vi "Test Parsing Simple Example Whlie Loop Some Operations 1.vi"() -> ()   [LabVIEW 2014]
uses:
  <vilib>/Utility/traverseref.llb/TRef TravTarget.ctl
  <vilib>/Utility/traverseref.llb/VI Scripting - Traverse.lvlib
panel:
  out "WhileLoop code chunks":T1
  out "Array 2":string[](array[string])
  out "error out":errorcluster
  out "SubVI C calls":string[](array[string])
  out "error wires info":T2
  in  "vi path":path=path "C:/Users/lubo/Documents/LabView/LabVIEW-Universal-Transcriptor/Test/Examples For Parsing/Example While Loop Some Operations 1.vi"
  # "This is here just for debug, for now I'm going to scan error wires and transcript VI on it to some C call functions."
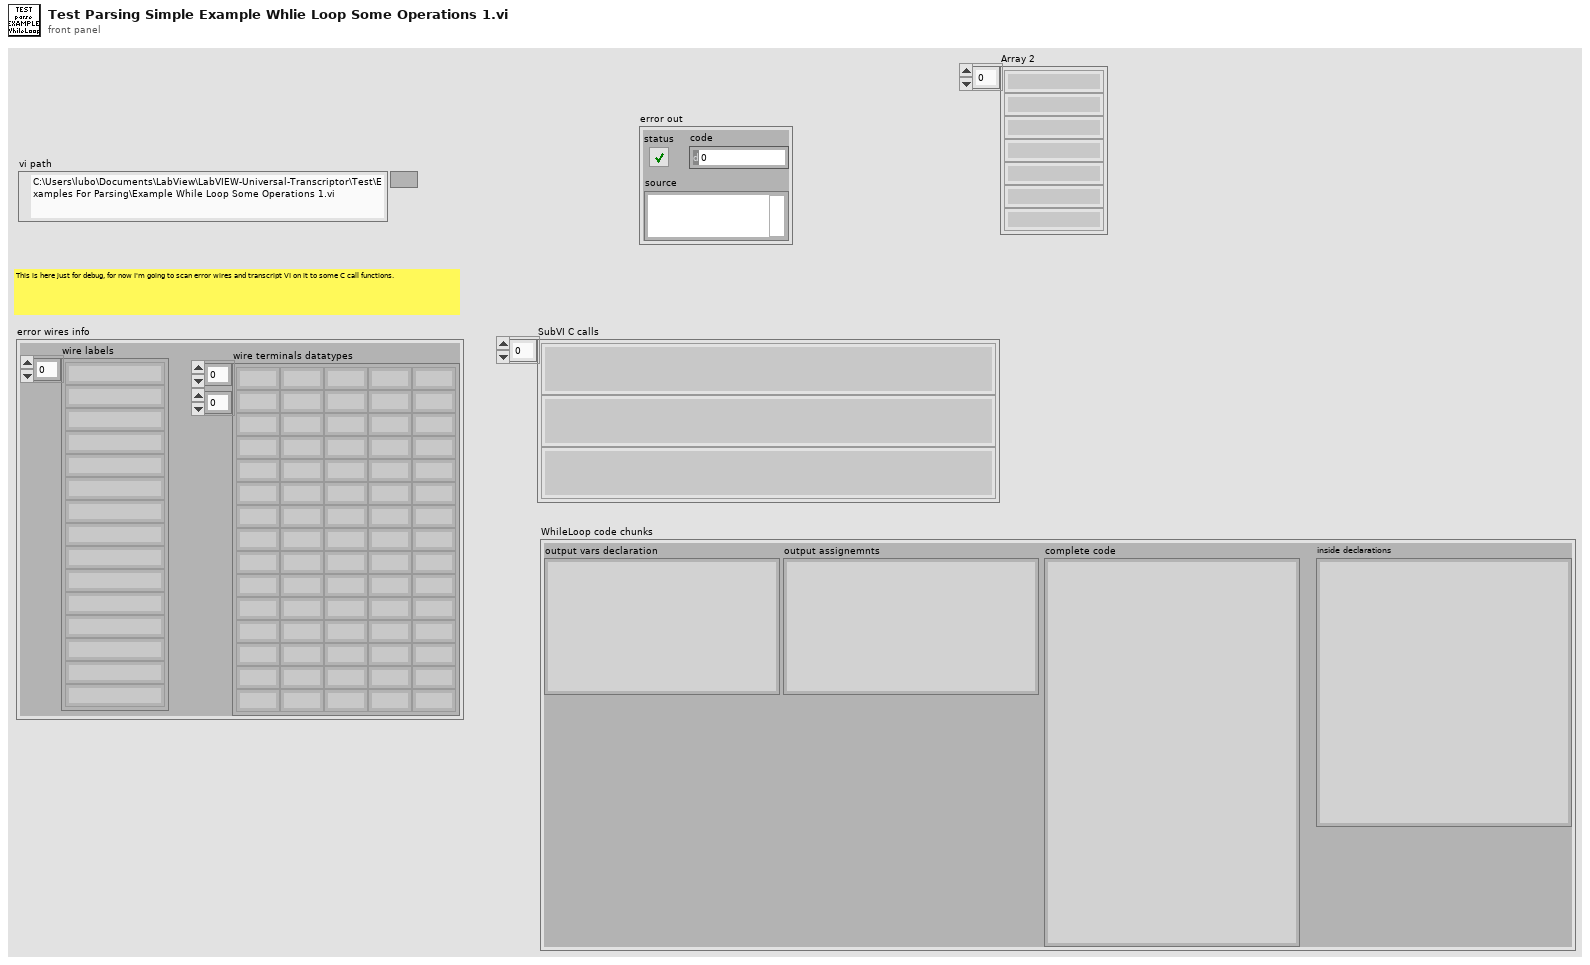
[diagram p1: front panel]
types:
  T1 = cluster{"output vars declaration":string, "output assignemnts":string, "complete code":string, "inside declarations":string}
  T2 = cluster{"wire labels":string[], "wire terminals datatypes":string[][]}
  T3 = typedef "TRef TravTarget.ctl" = enum16{"FP", "BD", "Other"}
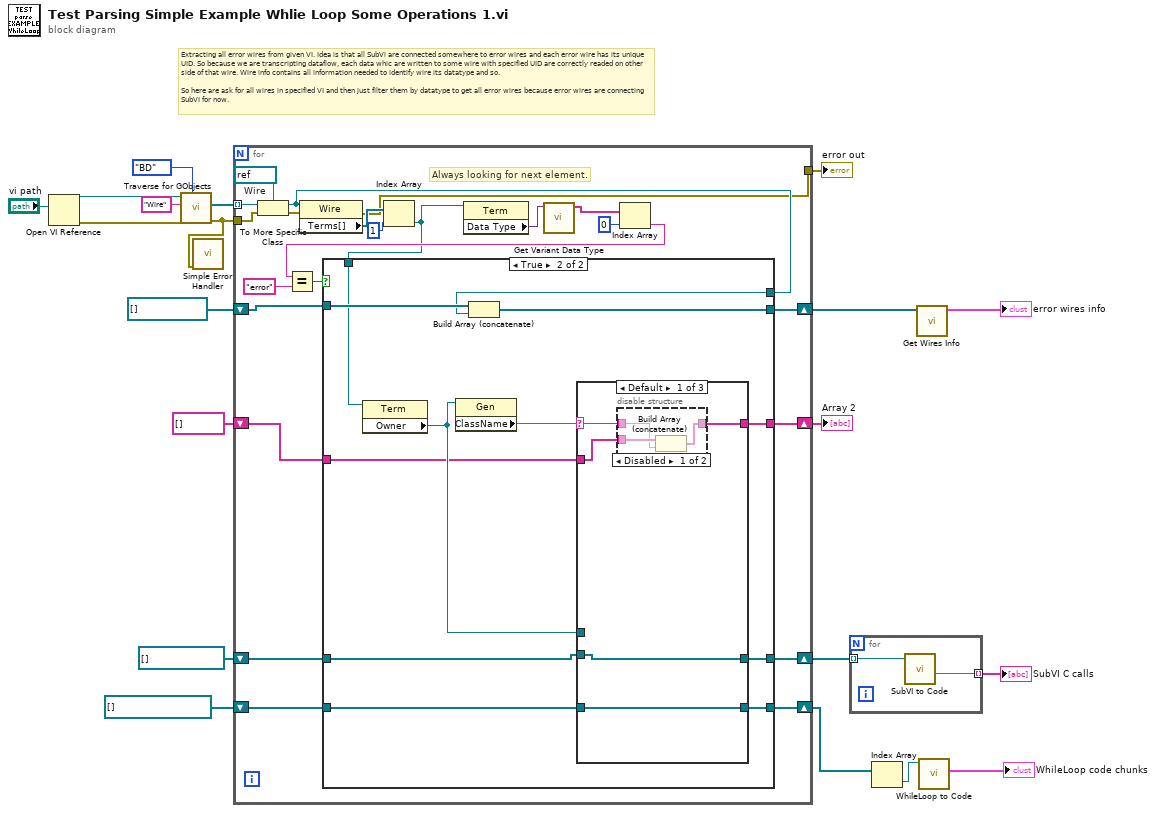
[diagram p0: block diagram]
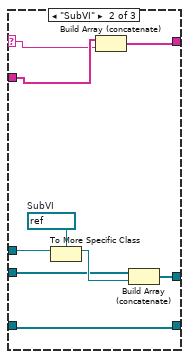
[diagram p4: hidden frame]
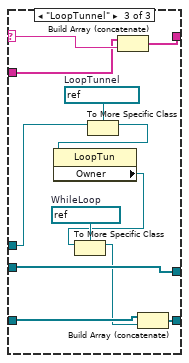
[diagram p5: hidden frame]
diagram:
  # "Extracting all error wires from given VI. Idea is that all SubVi are connected somewhere to error wires and each error wire has its unique UID. So because we are transcripting dataflow, each data whic are written to some wire with specified UID are correctly readed on other side of that wire. Wire info contains all information needed to identify wire its datatype and so.\n\nSo here are ask for all wires in specified VI and then just filter them by datatype to get all error wires because error wires are connecting SubVI for now."
  n1 = Open VI Reference(vi path="vi path") -> (vi reference=w19:refnum<vi>, error out=w16:errorcluster)  [unwired: 5 in]
  n2 = call <vilib>:"Traverse for GObjects.vi"("Traverse Target"=TRef_TravTarget."BD", "error in (no error)"=w16, "Class Name"="Wire", "VI Refnum"=w19) -> ("error out"=w8:errorcluster, "References"=w15:refnum<vi>[])  [unwired: 4 in, 2 out]
  n3 = call <vilib>:"Simple Error Handler.vi"("error in (no error)"=w8) -> ()  [unwired: 4 in, 5 out]
  n4 = for {
    tunnel: w15 -> [w33] mode=indexing
    tunnel: w8 -> [w43]
    shift-right: [w31] -> w13
    shift-left: refnum<vi>[] [] -> [w30]
    shift-right: [w28] -> w10
    shift-left: refnum<vi>[] [] -> [w27]
    tunnel: [w25] -> w9
    shift-right: [w23] -> w5
    shift-left: refnum<vi>[] [] -> [w24]
    shift-right: [w22] -> w3
    shift-left: string[] [] -> [w21]
    w42 = refnum<vi> refnum  # Wire
    # "Always looking for next element."
    n5 = To More Specific Class(target class=w42, reference=w33, error in=w43) -> (specific class reference=w32:refnum<vi>, error out=w41:errorcluster)
    n6 = property class="Wire"(reference=w32, error in=w41) -> (error out=w25:errorcluster, "Terms[]"=w40:refnum<vi>[])  [unwired: 1 out]
    n7 = Index Array(array=w40, index=1) -> (element=w26:refnum<vi>)
    n8 = property class="Term"(reference=w26) -> ("Data Type"=w39:variant)  [unwired: 1 in, 2 out]
    n9 = call "Get Variant Data Type.vi"("variant"=w39) -> ("Data Type"=w38:string[])  [unwired: 10 in]
    n10 = Index Array(array=w38, index=0) -> (element=w36:string)
    n11 = Equal?(x=w36, y="error") -> (x = y?=w29:bool)
    n12 = case shown="True" w29 {
      tunnel: w32 -> [_ w53]
      tunnel: [w47 w59] -> w31
      tunnel: w30 -> [w47 w58]
      tunnel: [w46 w56] -> w28
      tunnel: w27 -> [w46 w55]
      tunnel: w26 -> [_ w54]
      tunnel: w24 -> [w45 w51]
      tunnel: [w45 w50] -> w23
      tunnel: [w44 w49] -> w22
      tunnel: w21 -> [w44 w48]
      frame False {
      }
      frame True {
        n13 = property class="Term"(reference=w54) -> ("Owner"=w57:refnum<vi>)  [unwired: 1 in, 2 out]
        n14 = property class="Gen"(reference=w57) -> ("ClassName"=w52:string)  [unwired: 1 in, 2 out]
        n15 = Build Array (concatenate)(w58, w53) -> (w59:refnum<vi>[])
        n16 = case shown="Default" w52 {
          selector: w52 -> [w61 w70 w83]
          tunnel: w57 -> [_ w76 w80]
          tunnel: [w64 w73 w88] -> w56
          tunnel: w55 -> [w64 w74 w88]
          tunnel: w51 -> [w63 w72 w86]
          tunnel: [w63 w72 w87] -> w50
          tunnel: [w60 w69 w84] -> w49
          tunnel: w48 -> [w62 w71 w82]
          frame Default {
            n17 = disable-structure shown="Disabled" {
              disable-tunnel: w62 -> [w67 w68]
              disable-tunnel: w61 -> [w66 _]
              disable-tunnel: [w65 w68] -> w60
              frame Disabled {
                n18 = Build Array (concatenate)(w67, w66) -> (w65:string[])
              }
              frame Enabled {
              }
            }
          }
          frame "SubVI" {
            w77 = refnum<vi> refnum  # SubVI
            n19 = To More Specific Class(target class=w77, reference=w76) -> (specific class reference=w75:refnum<vi>)  [unwired: 1 in, 1 out]
            n20 = Build Array (concatenate)(w71, w70) -> (w69:string[])
            n21 = Build Array (concatenate)(w74, w75) -> (w73:refnum<vi>[])
          }
          frame "LoopTunnel" {
            w81 = refnum<vi> refnum  # LoopTunnel
            w89 = refnum<vi> refnum  # WhileLoop
            n22 = To More Specific Class(target class=w81, reference=w80) -> (specific class reference=w79:refnum<vi>)  [unwired: 1 in, 1 out]
            n23 = property class="LoopTun"(reference=w79) -> ("Owner"=w78:refnum<vi>)  [unwired: 1 in, 2 out]
            n24 = To More Specific Class(target class=w89, reference=w78) -> (specific class reference=w85:refnum<vi>)  [unwired: 1 in, 1 out]
            n25 = Build Array (concatenate)(w82, w83) -> (w84:string[])
            n26 = Build Array (concatenate)(w86, w85) -> (w87:refnum<vi>[])
          }
        }
      }
    }
  }
  "error out" <- w9
  "Array 2" <- w3
  n27 = for {
    tunnel: w10 -> [w91] mode=indexing
    tunnel: [w90] -> w6 mode=indexing
    n28 = call "SubVI to Code.vi"("reference"=w91) -> ("SubVI C call"=w90:string)  [unwired: 8 in, 2 out]
  }
  "SubVI C calls" <- w6
  n29 = Index Array(array=w5) -> (element=w2:refnum<vi>)  [unwired: 1 in]
  n30 = call "Get Wires Info.vi"("connected\nwires refs."=w13) -> ("output cluster 2"=→"error wires info":T2)  [unwired: 10 in]
  n31 = call "WhileLoop to Code.vi"("WhileLoop ref"=w2) -> ("WhileLoop code chunks"=→"WhileLoop code chunks":T1)  [unwired: 8 in, 2 out]
